vi "Actor Core.vi"(8 "error in":errorcluster, 11 "File Explorer In":refnum<class "File Explorer.lvclass">) -> (0 "error out":errorcluster, 3 "Actor out":refnum<class "Actor.lvclass">)   [LabVIEW 2017, in "File Explorer.lvlib" / "File Explorer.lvclass"]
doc: "(<B>Filename</B>: Actor Framework.lvlib:Actor.lvclass:Actor Core.vi)\n\nReceives messages to the actor, reacts to them, and initiates any error handling that may shut the actor down.\n\nDescendant classes may override this VI to append parallel tasks for the actor to complete while it handles messages. Overrides use the Call Parent Method node.\n\n<License>\nCopyright © 2017 Composed Systems, LLC | All rights reserved\nwww.composed.io\n\nAuthor: Ethan Stern <ethan.stern@composed.io>\n\nThis software is provided \"AS IS\" WITHOUT WARRANTIES, either express or implied, AND IS FOR EDUCATIONAL PURPOSES ONLY.\n</License>"
uses:
  <vilib>/gpm_packages/@cs/file-explorer-extension/Source/File Explorer/File Explorer/File Explorer.lvclass
  C:/Program Files/National Instruments/LabVIEW 2017/vi.lib/gpm_packages/@cs/mva-viewable/Source/ActorEvents/IEventAggregator/IEventAggregator.lvclass
  C:/Program Files/National Instruments/LabVIEW 2017/vi.lib/ActorFramework/Actor/Actor.lvclass
  <vilib>/ActorFramework/Actor/Actor.lvclass
  <vilib>/event_ctls.llb/lveventtype.ctl
  <vilib>/gpm_packages/@cs/file-explorer-extension/Source/File Explorer/File Explorer Event Filter/File Explorer Event Filter.lvclass
  C:/Program Files/National Instruments/LabVIEW 2017/vi.lib/gpm_packages/@cs/mva-viewable/Source/ActorEvents/IEventFilter/IEventFilter.lvclass
  <vilib>/gpm_packages/@cs/file-explorer-extension/Source/File Explorer/File Explorer/File Explorer.lvclass/File Explorer.ctl
  <vilib>/ActorFramework/Actor/Actor.lvclass/Actor.ctl
  <vilib>/ActorFramework/Message Enqueuer/Message Enqueuer.lvclass/Message Enqueuer.ctl
  <vilib>/gpm_packages/@cs/file-explorer-extension/Source/File Explorer/File Explorer Event Filter/File Explorer Event Filter.lvclass/File Explorer Event Filter.ctl
  <vilib>/ActorFramework/Message Enqueuer/Init from Existing Queue.vi
  <vilib>/ActorFramework/Message Enqueuer/Message Enqueuer.lvclass
  <vilib>/gpm_packages/@cs/mva-viewable/Source/IViewable/IViewable/IViewable.lvclass
  <vilib>/gpm_packages/@cs/mva-viewable/Source/ActorEvents/IEventAggregator/IEventAggregator.lvclass
  <vilib>/gpm_packages/@cs/mva-viewable/Source/ActorEvents/IEventFilter/IEventFilter.lvclass
  <vilib>/gpm_packages/@cs/file-explorer-extension/Source/File Explorer/File Explorer Messages/Handle Drag Starting Msg/Handle Drag Starting Msg.lvclass
  <vilib>/gpm_packages/@cs/file-explorer-extension/Source/File Explorer/File Explorer Messages/Handle Activate Menu On Tree Item Msg/Handle Activate Menu On Tree Item Msg.lvclass
panel:
  in  "Tree":string(tree)
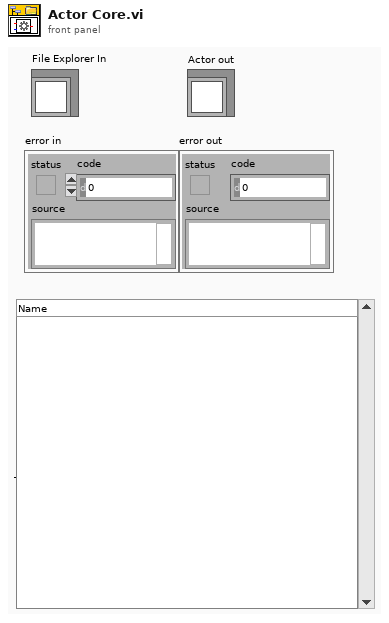
[diagram p1: front panel]
types:
  T1 = typedef "lveventtype.ctl" = enum32{"Null", "Timeout", "Annotation Menu Selection", "Annotation Menu Selection?", "App Instance Close", "App Instance Close?", "Autoscale Range Change", "Bookmark Info Change", "Cell Edit", "Cell Edit?", "Cursor Grab", "Cursor Grab?", "Cursor Menu Selection", "Cursor Menu Selection?", "Cursor Move", "Cursor Release", "Data Change", "Direction Change", "Display State Change", "Drag Ended", "Drag Enter", "Drag Leave", "Drag Over", "Drag Source Update", "Drag Starting", "Drag Starting?", "Drop", "Exec State Change", "Key Down", "Key Down?", "Key Repeat", "Key Repeat?", "Key Up", "Listbox Double Click", "Menu Activation?", "Menu Selection (App)", "Menu Selection? (App)", "Menu Selection (User)", "Mouse Down", "Mouse Down?", "Mouse Enter", "Mouse Leave", "Mouse Move", "Mouse Up", "Mouse Wheel", "NI Security User Change (App)", "Pane Size", "Panel Close", "Panel Close?", "Panel Resize", "Plot Attribute Change", "Scale Range Change", "Shortcut Menu Activation?", "Shortcut Menu Selection (App)", "Shortcut Menu Selection? (App)", "Shortcut Menu Selection (User)", "Tree Double Click", "Tree Drag", "Tree Drag?", "Tree Drop", "Tree Drop?", "Tree Item Close", "Tree Item Close?", "Tree Item Open", "Tree Item Open?", "User Event", "Value Change"}
  T2 = typedef "ActorEvents.lvlib/IEventFilter.lvclass/EventFilter Reference.ctl" = refnum<data-value>
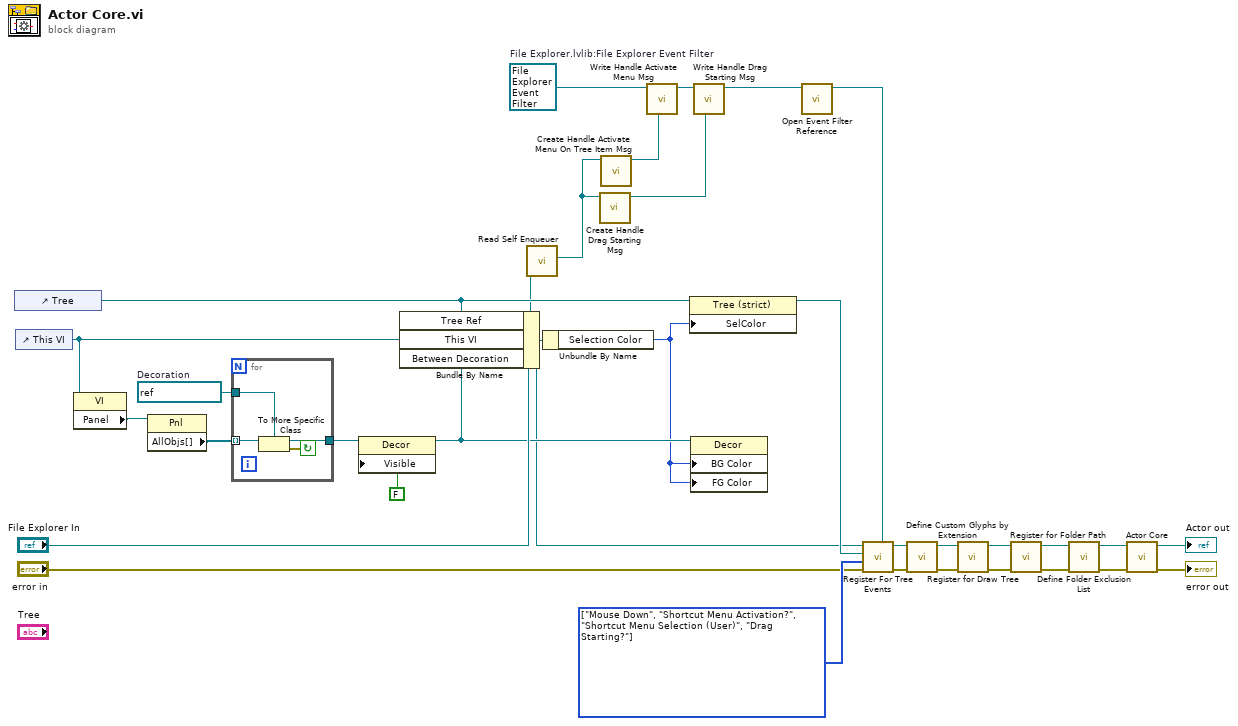
[diagram p0: block diagram]
diagram:
  w14 = refnum<vi> refnum  # Decoration
  w22 = refnum<class "File Explorer Event Filter.lvclass"> refnum  # File Explorer.lvlib:File Explorer Event Filter
  w23 = T1[] [enum."Mouse Down", enum."Shortcut Menu Activation?", enum."Shortcut Menu Selection (User)", enum."Drag Starting?"] items=["Null", "Timeout", "Annotation Menu Selection", "Annotation Menu Selection?", "App Instance Close", "App Instance Close?", "Autoscale Range Change", "Bookmark Info Change", "Cell Edit", "Cell Edit?", "Cursor Grab", "Cursor Grab?", "Cursor Menu Selection", "Cursor Menu Selection?", "Cursor Move", "Cursor Release", "Data Change", "Direction Change", "Display State Change", "Drag Ended", "Drag Enter", "Drag Leave", "Drag Over", "Drag Source Update", "Drag Starting", "Drag Starting?", "Drop", "Exec State Change", "Key Down", "Key Down?", "Key Repeat", "Key Repeat?", "Key Up", "Listbox Double Click", "Menu Activation?", "Menu Selection (App)", "Menu Selection? (App)", "Menu Selection (User)", "Mouse Down", "Mouse Down?", "Mouse Enter", "Mouse Leave", "Mouse Move", "Mouse Up", "Mouse Wheel", "NI Security User Change (App)", "Pane Size", "Panel Close", "Panel Close?", "Panel Resize", "Plot Attribute Change", "Scale Range Change", "Shortcut Menu Activation?", "Shortcut Menu Selection (App)", "Shortcut Menu Selection? (App)", "Shortcut Menu Selection (User)", "Tree Double Click", "Tree Drag", "Tree Drag?", "Tree Drop", "Tree Drop?", "Tree Item Close", "Tree Item Close?", "Tree Item Open", "Tree Item Open?", "User Event", "Value Change"] ("Registration Types")
  n1 = control-ref of="Tree"() -> (w10:refnum<vi>)
  n2 = control-ref of="This VI"() -> (w11:refnum<vi>)
  n3 = property class="VI"(reference=w11) -> ("Panel"=w16:refnum<vi>)  [unwired: 1 in, 2 out]
  n4 = property class="Pnl"(reference=w16) -> ("AllObjs[]"=w15:refnum<vi>[])  [unwired: 1 in, 2 out]
  n5 = for {
    tunnel: w15 -> [w37] mode=indexing
    tunnel: w14 -> [w36]
    tunnel: [w34] -> w13
    stop <- w35 continue-if-true
    n6 = To More Specific Class(target class=w36, reference=w37) -> (specific class reference=w34:refnum<vi>, error out=w35:errorcluster)  [unwired: 1 in]
  }
  n7 = property class="Decor"(reference=w13, "Visible"=FALSE) -> (reference out=w8:refnum<vi>)  [unwired: 1 in, 1 out]
  n8 = Bundle By Name(cluster="File Explorer In", "Tree Ref"=w10, "This VI"=w11, "Between Decoration"=w8) -> (w7:refnum<class "File Explorer.lvclass">)
  n9 = call <vilib>:"Read Self Enqueuer.vi"("Actor"=w7) -> ("Self Enqueuer"=w2:refnum<class "Message Enqueuer.lvclass">)  [unwired: 10 in]
  n10 = Unbundle By Name(w7) -> ("Selection Color"=w6:u32)
  n11 = call <vilib>:"Create Handle Drag Starting Msg.vi"("Return Enqueuer"=w2) -> ("Handle Drag Starting Msg out"=w3:refnum<class "Handle Drag Starting Msg.lvclass">)  [unwired: 10 in]
  n12 = call <vilib>:"Create Handle Activate Menu On Tree Item Msg.vi"("Return Enqueuer"=w2) -> ("Handle Activate Menu On Tree Item Msg out"=w1:refnum<class "Handle Activate Menu On Tree Item Msg.lvclass">)  [unwired: 10 in]
  n13 = call <vilib>:"Write Handle Activate Menu Msg.vi"("Handle Activate Menu On Tree Item Msg"=w1, "File Explorer Event Filter in"=w22) -> ("File Explorer Event Filter out"=w5:refnum<class "File Explorer Event Filter.lvclass">)  [unwired: 9 in]
  n14 = property class="Tree (strict)"(reference=w10, "SelColor"=w6) -> (reference out=w9:refnum<vi>)  [unwired: 1 in, 1 out]
  n15 = property class="Decor"(reference=w8, "BG Color"=w6, "FG Color"=w6) -> ()  [unwired: 1 in, 2 out]
  n16 = call <vilib>:"Write Handle Drag Starting Msg.vi"("Handle Drag Starting Msg"=w3, "File Explorer Event Filter in"=w5) -> ("File Explorer Event Filter out"=w4:refnum<class "File Explorer Event Filter.lvclass">)  [unwired: 9 in]
  n17 = call <vilib>:"Open Event Filter Reference.vi"("IEventFilter in"=w4) -> ("IEventFilter Reference"=w24:T2)  [unwired: 9 in, 1 out]
  n18 = call <vilib>:"Register For Tree Events.vi"("EventFilter Reference"=w24, "error in (no error)"="error in", "Registration Types"=w23, "Tree Refnum"=w9, "IEventAggregator In"=w7) -> ("error out"=w26:errorcluster, "IEventAggregator Out"=w25:refnum<class "File Explorer.lvclass">)  [unwired: 5 in]
  n19 = call-dynamic "Define Custom Glyphs by Extension.vi"("error in (no error)"=w26, "File Explorer in"=w25) -> ("error out"=w18:errorcluster, "File Explorer out"=w20:refnum<class "File Explorer.lvclass">)  [unwired: 8 in]
  n20 = call-dynamic "Register for Draw Tree.vi"("error in (no error)"=w18, "File Explorer in"=w20) -> ("error out"=w17:errorcluster, "File Explorer out"=w19:refnum<class "File Explorer.lvclass">)  [unwired: 8 in]
  n21 = call-dynamic "Register for Folder Path.vi"("error in (no error)"=w17, "File Explorer in"=w19) -> ("error out"=w28:errorcluster, "File Explorer out"=w30:refnum<class "File Explorer.lvclass">)  [unwired: 8 in]
  n22 = call-dynamic "Define Folder Exclusion List.vi"("error in (no error)"=w28, "File Explorer in"=w30) -> ("error out"=w27:errorcluster, "File Explorer out"=w29:refnum<class "File Explorer.lvclass">)  [unwired: 8 in]
  n23 = call-parent "Actor Core.vi"("error in"=w27, "IViewable In"=w29) -> ("error out"=→"error out":errorcluster, "Actor out"=→"Actor out":refnum<class "Actor.lvclass">)  [unwired: 8 in]
